vi "controlChainGain.vi"(7 "Set":bool, 8 "error in":errorcluster, 9 "gainconfig":enum16{"0 dB", "-10 dB", "-15 dB", "-20 dB"}(ring), 10 "axis in":u8, 11 "connection ID":i32) -> (0 "error out":errorcluster, 1 "gainconfig out":enum16{"0 dB", "-10 dB", "-15 dB", "-20 dB"}(ring), 2 "axis out":u8, 3 "connection ID":i32)   [LabVIEW 2016]
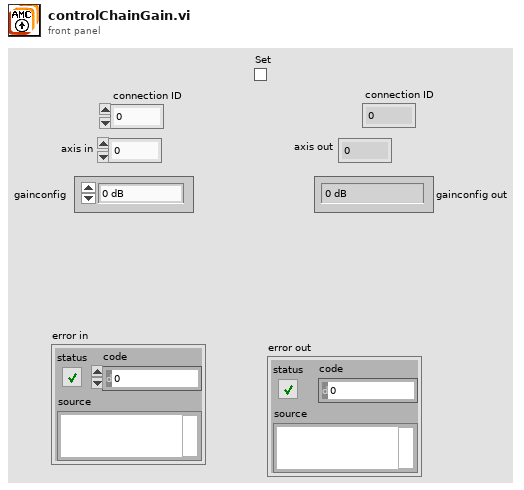
[diagram p1: front panel]
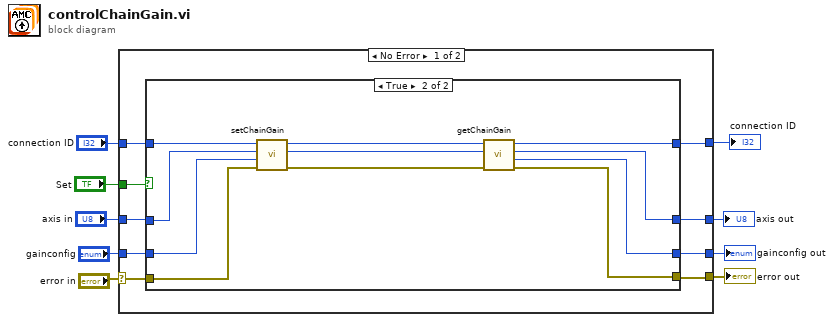
[diagram p0: block diagram]
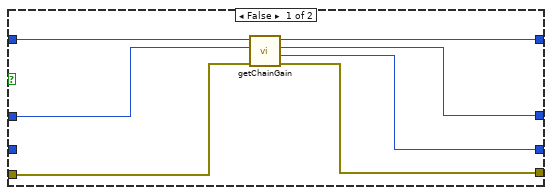
[diagram p2: hidden frame]
diagram:
  n1 = case shown="No Error" "error in" {
    selector: "error in" -> [w14 w40]
    tunnel: "axis in" -> [w16 w39]
    tunnel: [w11 w40] -> w8
    tunnel: [w12 w39] -> w7
    tunnel: "gainconfig" -> [w15 w37]
    tunnel: "Set" -> [w17 _]
    tunnel: [w13 w38] -> w4
    tunnel: "connection ID" -> [w18 w38]
    tunnel: [w10 w37] -> w1
    frame No Error {
      n2 = case shown="True" w17 {
        tunnel: [w24 w31] -> w13
        tunnel: w18 -> [w25 w36]
        tunnel: w16 -> [w21 w35]
        tunnel: [w20 w28] -> w12
        tunnel: [w22 w26] -> w11
        tunnel: w15 -> [_ w33]
        tunnel: w14 -> [w23 w34]
        tunnel: [w19 w27] -> w10
        frame False {
          n3 = call "getChainGain.vi"("error in"=w23, "axis"=w21, "connection ID"=w25) -> ("error out"=w22:errorcluster, "gaincoeff"=w19:i32, "axis_out"=w20:i32, "connection ID"=w24:i32)  [unwired: 5 in]
        }
        frame True {
          n4 = call "setChainGain.vi"("error in"=w34, "gainconfig"=w33, "axis"=w35, "connection ID"=w36) -> ("error out"=w30:errorcluster, "axis_out"=w29:i32, "connection ID"=w32:i32)  [unwired: 5 in]
          n5 = call "getChainGain.vi"("error in"=w30, "axis"=w29, "connection ID"=w32) -> ("error out"=w26:errorcluster, "gaincoeff"=w27:i32, "axis_out"=w28:i32, "connection ID"=w31:i32)  [unwired: 5 in]
        }
      }
    }
    frame Error {
    }
  }
  "error out" <- w8
  "axis out" <- w7
  "connection ID" <- w4
  "gainconfig out" <- w1
